vi "validateScheduler.vi"(9 "Constraints":T1, 10 "Schedule":T2(array[cluster])) -> (1 "Invalid Input":bool, 2 "Valid Input":bool)   [LabVIEW 2018]
panel:
  out "Setpoint Array":dbl[](array[numeric])
  out "Frequency Array":dbl[](array[numeric])
  out "Time Array":dbl[](array[numeric])
  out "Max Rate":dbl
  out "Min Value":dbl
  out "Max Value":dbl
  # "For Debugging: Constraints and Variables"
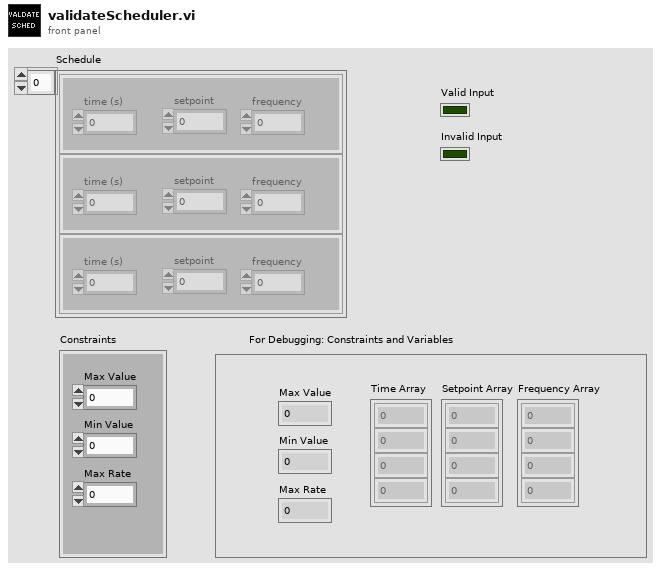
[diagram p1: front panel]
types:
  T1 = cluster{"Max Value":dbl, "Min Value":dbl, "Max Rate":dbl}
  T2 = cluster{"time (s)":dbl, "setpoint ":dbl, "frequency":dbl}[]
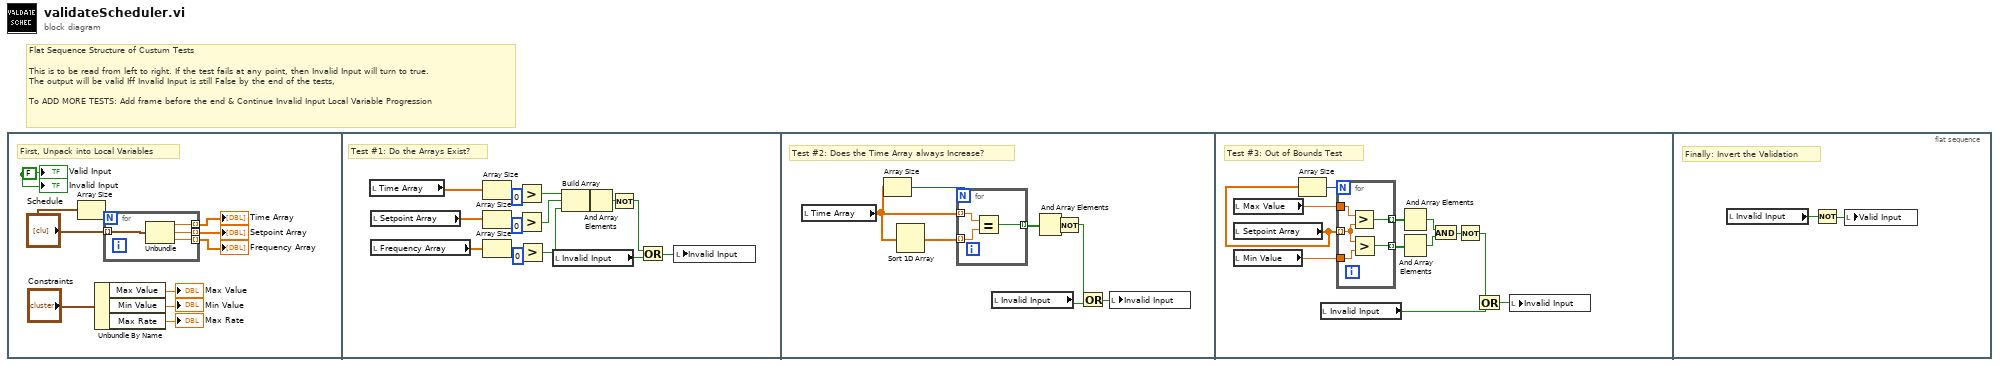
[diagram p0: block diagram]
diagram:
  # "Flat Sequence Structure of Custum Tests\n\nThis is to be read from left to right. If the test fails at any point, then Invalid Input will turn to true.\nThe output will be valid Iff Invalid Input is still False by the end of the tests,\n\nTo ADD MORE TESTS: Add frame before the end & Continue Invalid Input Local Variable Progression"
  n1 = flat-sequence {
    frame #0 {
      w10 = FALSE
      # "First, Unpack into Local Variables"
      n2 = Array Size(array="Schedule") -> (size(s)=w5:i32)
      n3 = Unbundle By Name("Constraints") -> ("Max Value"=→"Max Value":dbl, "Min Value"=→"Min Value":dbl, "Max Rate"=→"Max Rate":dbl)
      n4 = for {
        N: w5 -> [_]
        tunnel: "Schedule" -> [w14] mode=indexing
        tunnel: [w13] -> w8 mode=indexing
        tunnel: [w12] -> w7 mode=indexing
        tunnel: [w11] -> w9 mode=indexing
        n5 = Unbundle(w14) -> ("time (s)"=w13:dbl, "setpoint"=w12:dbl, "frequency"=w11:dbl)
      }
      "Time Array" <- w8
      "Frequency Array" <- w9
      "Setpoint Array" <- w7
      "Valid Input" <- w10
      "Invalid Input" <- w10
    }
    frame #1 {
      # "Test #1: Do the Arrays Exist?"
      n6 = local read "Time Array"() -> (w31:dbl[])
      n7 = local read "Setpoint Array"() -> (w30:dbl[])
      n8 = local read "Frequency Array"() -> (w29:dbl[])
      n9 = Array Size(array=w31) -> (size(s)=w22:i32)
      n10 = Array Size(array=w30) -> (size(s)=w23:i32)
      n11 = Array Size(array=w29) -> (size(s)=w24:i32)
      n12 = Greater?(x=w22, y=0) -> (0:w21:bool)
      n13 = Greater?(x=w23, y=0) -> (0:w20:bool)
      n14 = Greater?(x=w24, y=0) -> (0:w19:bool)
      n15 = local read "Invalid Input"() -> (w18:bool)
      n16 = Build Array(w21, w20, w19) -> (w28:bool[])
      n17 = And Array Elements(Boolean array=w28) -> (logical AND=w15:bool)
      n18 = Not(x=w15) -> (.not. x?=w16:bool)
      n19 = Or(x=w16, y=w18) -> (x .or. y?=w17:bool)
      n20 = local write "Invalid Input"(w17) -> ()
    }
    frame #2 {
      # "Test #2: Does the Time Array always Increase?"
      n21 = local read "Time Array"() -> (w38:dbl[])
      n22 = Array Size(array=w38) -> (size(s)=w39:i32)
      n23 = Sort 1D Array(array=w38) -> (sorted array=w37:dbl[])
      n24 = for {
        N: w39 -> [_]
        tunnel: w38 -> [w42] mode=indexing
        tunnel: w37 -> [w41] mode=indexing
        tunnel: [w40] -> w36 mode=indexing
        n25 = Equal?(x=w42, y=w41) -> (x = y?=w40:bool)
      }
      n26 = local read "Invalid Input"() -> (w34:bool)
      n27 = And Array Elements(Boolean array=w36) -> (logical AND=w33:bool)
      n28 = Not(x=w33) -> (.not. x?=w32:bool)
      n29 = Or(x=w32, y=w34) -> (x .or. y?=w35:bool)
      n30 = local write "Invalid Input"(w35) -> ()
    }
    frame #3 {
      # "Test #3: Out of Bounds Test"
      n31 = local read "Max Value"() -> (w52:dbl)
      n32 = local read "Setpoint Array"() -> (w51:dbl[])
      n33 = local read "Min Value"() -> (w53:dbl)
      n34 = Array Size(array=w51) -> (size(s)=w54:i32)
      n35 = local read "Invalid Input"() -> (w45:bool)
      n36 = for {
        N: w54 -> [_]
        tunnel: w53 -> [w57]
        tunnel: w52 -> [w59]
        tunnel: w51 -> [w58] mode=indexing
        tunnel: [w56] -> w50 mode=indexing
        tunnel: [w55] -> w49 mode=indexing
        n37 = Greater?(x=w59, y=w58) -> (0:w56:bool)
        n38 = Greater?(x=w58, y=w57) -> (0:w55:bool)
      }
      n39 = And Array Elements(Boolean array=w50) -> (logical AND=w47:bool)
      n40 = And Array Elements(Boolean array=w49) -> (logical AND=w48:bool)
      n41 = And(x=w47, y=w48) -> (x .and. y?=w44:bool)
      n42 = Not(x=w44) -> (.not. x?=w43:bool)
      n43 = Or(x=w43, y=w45) -> (x .or. y?=w46:bool)
      n44 = local write "Invalid Input"(w46) -> ()
    }
    frame #4 {
      # "Finally: Invert the Validation"
      n45 = local read "Invalid Input"() -> (w61:bool)
      n46 = Not(x=w61) -> (.not. x?=w60:bool)
      n47 = local write "Valid Input"(w60) -> ()
    }
  }
